vi "Step_3_Ans_For_loop_PS.vi"   [LabVIEW 2012]
types:
  T1 = typedef "BotSpeak_Control.ctl" = cluster{"Address":string, "Reply EOF":string, "Hardware":string, "Retries":i8, "Timeout":i32}
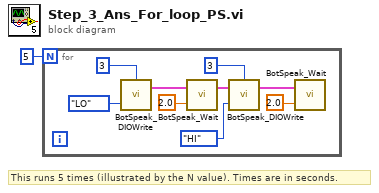
[diagram p0: block diagram]
diagram:
  # "This runs 5 times (illustrated by the N value). Times are in seconds."
  n1 = for {
    N: 5 -> [_]
    n2 = call <userlib>:"BotSpeak_DIOWrite.vi"("State"=enum32{"LO", "HI"}."LO", "DIO Line"=u32 3) -> ("Bot Settings"=w4:T1)  [unwired: 1 in, 1 out]
    n3 = call <userlib>:"BotSpeak_Wait.vi"("Wait (sec)"=2.0, "Bot Settings"=w4) -> ("Bot Settings"=w5:T1)  [unwired: 1 in]
    n4 = call <userlib>:"BotSpeak_DIOWrite.vi"("State"=enum32{"LO", "HI"}."HI", "Bot Settings"=w5, "DIO Line"=u32 3) -> ("Bot Settings"=w3:T1)  [unwired: 1 out]
    n5 = call <userlib>:"BotSpeak_Wait.vi"("Wait (sec)"=2.0, "Bot Settings"=w3) -> ()  [unwired: 1 in, 1 out]
  }
